vi "GageGlobals.vi"() -> ()   [LabVIEW 2022 SP3]
panel:
  in  "Shot Number":i32
  in  "Acq Vals 2":T1={"Sample Rate"=100000000.0, "Clock Mode"=enum."Internal", "Mode"="Dual", "Depth"=8192.0, "Segment Size"=8192.0, "Trigger Timeout"=1000000.0, "Trigger Holdoff"=0.0, "Trigger Delay"=0.0}
  out "Scope ID":refnum<visa-resource-name>
  out "amplitude (kV)":dbl=50.0 format="%.2f"
  in  "Avg Num":i32=1 min=1
  in  "c mm/mics":sgl=1.485
  in  "Additional dig delay (ms)":dbl format="%.2f"
  in  "Digitizer delay\n (ms)":dbl format="%.2f"
  in  "Samp Rate (Hz)":dbl
  in  "rf points per line":i32=2048
  in  "Ch Vals 2":T2(array[cluster])=[{"Coupling"="DC", "Diff. Input"=FALSE, "Direct-to-ADC"=FALSE, "Input Range"=2000, "Impedance"=1000000, "DC Offset"=0, "Filter(0)"=0}] {"Impedance" min=50 max=1000000 step=999950}
  in  "# Firings":u16=1 min=1
  in  "Trig Vals":T3(array[cluster])=[{"Slope"="Rising", "Level"=0, "Source"=0, "External Range"=2000, "External Coupling"="DC", "External Trigger"=FALSE, "Disable Trigger"=FALSE, "External Impedance"="HiZ"}] {"External Range" min=2000 max=10000 step=8000; "Level" min=-100 max=100; "Source" min=0 max=64 step=1}
  in  "Ch Vals 1":T2(array[cluster])=[{"Coupling"="DC", "Diff. Input"=FALSE, "Direct-to-ADC"=FALSE, "Input Range"=2000, "Impedance"=1000000, "DC Offset"=0, "Filter(0)"=0}] {"Impedance" min=50 max=1000000 step=999950}
  in  "Acq Vals 1":T1={"Sample Rate"=100000000.0, "Clock Mode"=enum."Internal", "Mode"="Dual", "Depth"=8192.0, "Segment Size"=8192.0, "Trigger Timeout"=1000000.0, "Trigger Holdoff"=0.0, "Trigger Delay"=0.0}
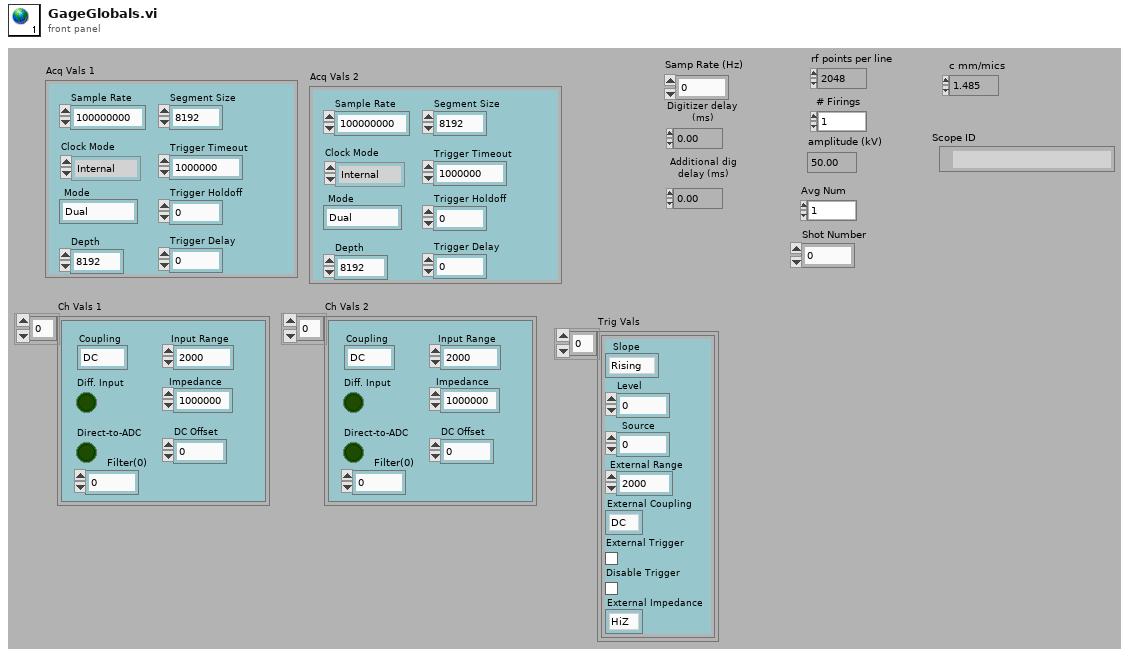
[diagram p1: front panel]
types:
  T1 = cluster{"Sample Rate":dbl, "Clock Mode":enum16{"Internal", "External", "Reference"}, "Mode":string, "Depth":dbl, "Segment Size":dbl, "Trigger Timeout":dbl, "Trigger Holdoff":dbl, "Trigger Delay":dbl}
  T2 = cluster{"Coupling":string, "Diff. Input":bool, "Direct-to-ADC":bool, "Input Range":i32, "Impedance":u32, "DC Offset":i32, "Filter(0)":u32}[]
  T3 = cluster{"Slope":string, "Level":i32, "Source":i32, "External Range":u32, "External Coupling":string, "External Trigger":bool, "Disable Trigger":bool, "External Impedance":string}[]
diagram:
